vi "Save Resource File.vi"(8 "error in (no error)":errorcluster, 9 "Path":path, 10 "File type":string, 11 "Resources":T1) -> (0 "error out":errorcluster)   [LabVIEW 2017]
uses:
  Resource Array.ctl
  Resource.ctl
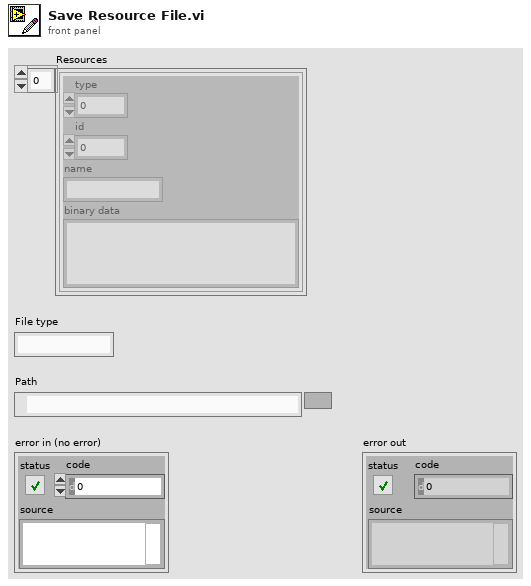
[diagram p1: front panel]
types:
  T1 = typedef "Resource Array.ctl" = T2[]
  T2 = typedef "Resource.ctl" = cluster{"type":u32, "id":i32, "name":string, "binary data":string}
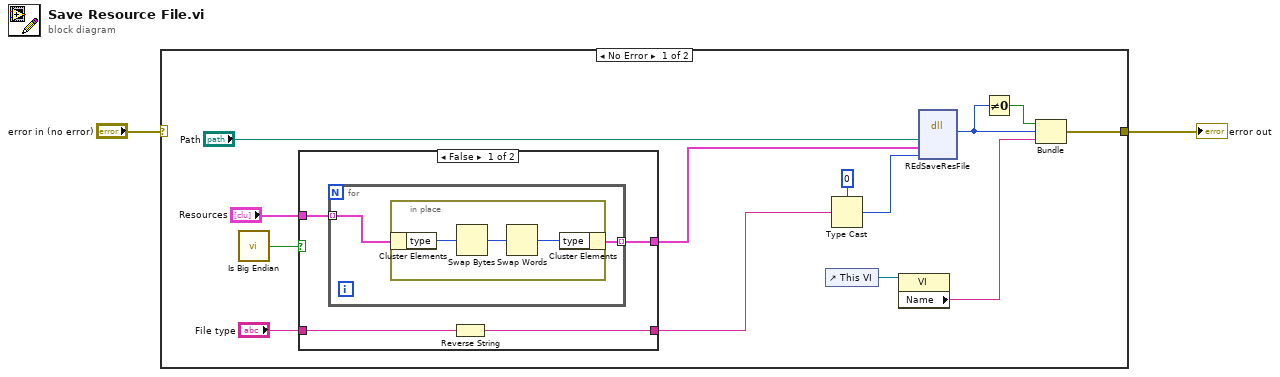
[diagram p0: block diagram]
diagram:
  n1 = case shown="No Error" "error in (no error)" {
    selector: "error in (no error)" -> [_ w27]
    tunnel: [w8 w27] -> w2
    frame No Error {
      n2 = call "Is Big Endian.vi"() -> ("big endian"=w3:bool)
      n3 = case shown="False" w3 {
        tunnel: "Resources" -> [w16 w26]
        tunnel: [w19 w26] -> w6
        tunnel: "File type" -> [w18 w25]
        tunnel: [w17 w25] -> w4
        frame False {
          n4 = for {
            tunnel: [w21] -> w19 mode=indexing
            tunnel: w16 -> [w20] mode=indexing
            n5 = in-place {
              n6 = in-place-cluster #1(w20) -> ("type"=w24:u32)
              n7 = Swap Bytes(anything=w24) -> (byte swapped=w23:u32)
              n8 = Swap Words(1:w23) -> (0:w22:u32)
              n9 = in-place-cluster #1("type"=w22) -> (w21:T2)
            }
          }
          n10 = Reverse String(1:w18) -> (0:w17:string)
        }
        frame True {
        }
      }
      n11 = control-ref of="This VI"() -> (w12:refnum<vi>)
      n12 = Type Cast(type=0, x=w4) -> (*(type *) &x=w14:i32)
      n13 = property class="VI"(reference=w12) -> ("Name"=w9:string)  [unwired: 1 in, 2 out]
      n14 = dll-call lib="LabVIEW" fn="REdSaveResFile"("Path", w6, w14) -> ("return type"=w10:i32)  [unwired: 6 in, 2 out]
      n15 = Not Equal To 0?(x=w10) -> (x != 0?=w11:bool)
      n16 = Bundle(w11, "return type"=w10, "Name"=w9) -> (w8:cluster{bool, "return type":i32, "Name":string})  [unwired: 1 in]
    }
    frame Error {
    }
  }
  "error out" <- w2
